vi "Arcade Close.vi"(11 "Arcade Drive":T1) -> ()   [LabVIEW 2013]
uses:
  Arcade Drive Ref.ctl
  <vilib>/Rock Robotics/WPI/MotorControl/WPI_MotorControlDeviceRef.ctl
  <vilib>/Rock Robotics/SystemInterfaces/Typedef/FPGA_TypedefDigitalModule.ctl
  <vilib>/Rock Robotics/SystemInterfaces/DIO/FPGA_DIOPWMChannel.ctl
  <vilib>/Rock Robotics/WPI/PWM/WPI_PWMDeadband.ctl
  <vilib>/Rock Robotics/WPI/CAN/Jaguar/SubVIs/WPI_CANJaguar_ControlMode.ctl
  <vilib>/Rock Robotics/WPI/PWM/WPI_PWMTransform_ConPane.ctl
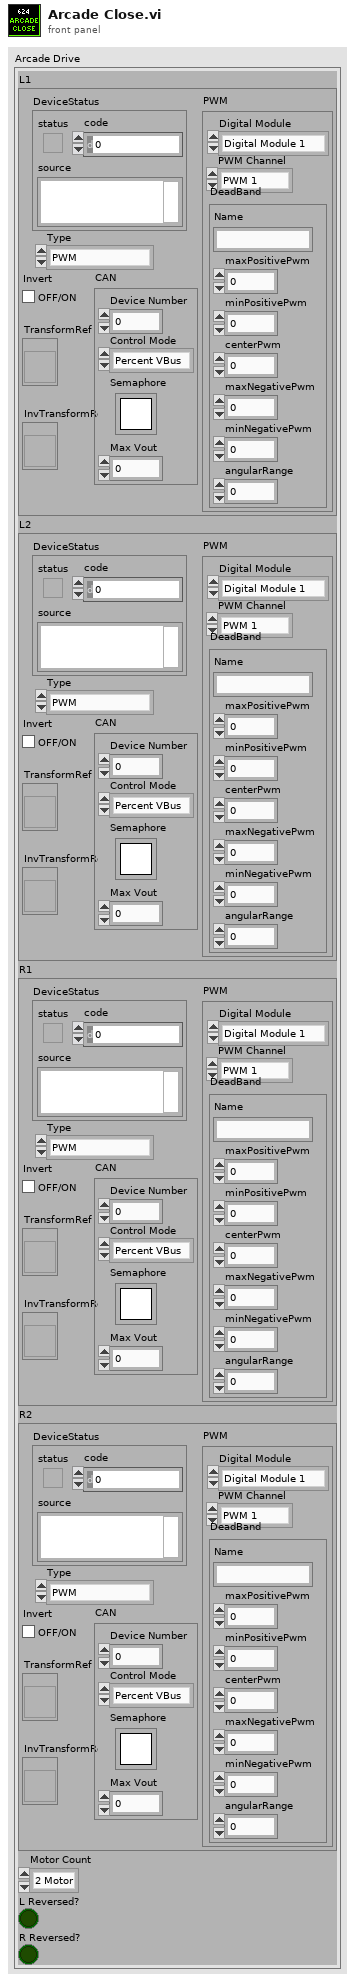
[diagram p1: front panel]
types:
  T1 = typedef "Arcade Drive Ref.ctl" = cluster{"L1":T2, "L2":T2, "R1":T2, "R2":T2, "Motor Count":enum16{"2 Motor", "4 Motor"}, "L Reversed?":bool, "R Reversed?":bool}
  T2 = typedef "WPI_MotorControlDeviceRef.ctl" = cluster{"DeviceStatus":errorcluster, "Type":enum16{"PWM", "CAN"}, "PWM":cluster{"Digital Module":T3, "PWM Channel":T4, "DeadBand":T5}, "CAN":cluster{"Device Number":u8, "Control Mode":T6, "Semaphore":T7, "Max Vout":dbl}, "Invert":bool, "TransformRef":T8, "InvTransformRef":T8}
  T3 = typedef "FPGA_TypedefDigitalModule.ctl" = enum16{"Digital Module 1", "Digital Module 2"}
  T4 = typedef "FPGA_DIOPWMChannel.ctl" = enum8{"PWM 1", "PWM 2", "PWM 3", "PWM 4", "PWM 5", "PWM 6", "PWM 7", "PWM 8", "PWM 9", "PWM 10", "Invalid"}
  T5 = typedef "WPI_PWMDeadband.ctl" = cluster{"Name":string, "maxPositivePwm":i32, "minPositivePwm":i32, "centerPwm":i32, "maxNegativePwm":i32, "minNegativePwm":i32, "angularRange":u16}
  T6 = typedef "WPI_CANJaguar_ControlMode.ctl" = enum8{"Percent VBus", "Current", "Speed", "Position", "Voltage"}
  T7 = typedef "Semaphore RefNum" = refnum<k1>
  T8 = typedef "WPI_PWMTransform_ConPane.ctl" = refnum<vi>
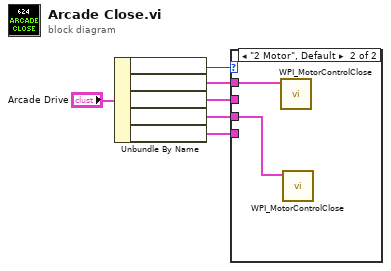
[diagram p0: block diagram]
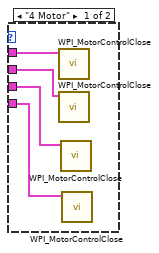
[diagram p2: hidden frame]
diagram:
  n1 = Unbundle By Name("Arcade Drive") -> (w5:enum16{"2 Motor", "4 Motor"}, w4:T2, w3:T2, w2:T2, w1:T2)
  n2 = case shown="\"2 Motor\", Default" w5 {
    tunnel: w4 -> [w10 w12]
    tunnel: w3 -> [w9 _]
    tunnel: w2 -> [w8 w11]
    tunnel: w1 -> [w7 _]
    frame "4 Motor" {
      n3 = call <vilib>:"WPI_MotorControlClose.vi"(11:w10) -> ()  [unwired: 10 in, 1 out]
      n4 = call <vilib>:"WPI_MotorControlClose.vi"(11:w9) -> ()  [unwired: 10 in, 1 out]
      n5 = call <vilib>:"WPI_MotorControlClose.vi"(11:w8) -> ()  [unwired: 10 in, 1 out]
      n6 = call <vilib>:"WPI_MotorControlClose.vi"(11:w7) -> ()  [unwired: 10 in, 1 out]
    }
    frame "2 Motor", Default {
      n7 = call <vilib>:"WPI_MotorControlClose.vi"(11:w12) -> ()  [unwired: 10 in, 1 out]
      n8 = call <vilib>:"WPI_MotorControlClose.vi"(11:w11) -> ()  [unwired: 10 in, 1 out]
    }
  }
